vi "queue priority list.vi"() -> ()   [LabVIEW 2018]
uses:
  Support/Message Queue/queue priority list.ctl
  Support/Message Queue/queue priority info.ctl
  Support/Message Queue/Message Queue.lvlib
panel:
  in  "message queue priority list":T1
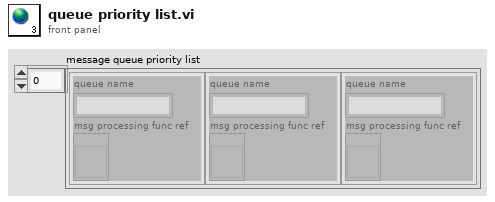
[diagram p1: front panel]
types:
  T1 = typedef "Message Queue.lvlib/queue priority list.ctl" = T2[]
  T2 = typedef "Message Queue.lvlib/queue priority info.ctl" = cluster{"queue name":string, "msg processing func ref":refnum<vi>}
diagram:
